vi "Test Enum.vi"(11 "Describe Variant Test in":refnum<class "Describe Variant Test.lvclass">) -> (0 "error out":errorcluster, 3 "Describe Variant Test out":refnum<class "Describe Variant Test.lvclass">)   [LabVIEW 2020, in "Describe Variant Test.lvclass"]
uses:
  Describe Variant Test.lvclass
  C:/Program Files (x86)/National Instruments/LabVIEW 2020/vi.lib/Astemes/LUnit/Test Case.lvclass
  <vilib>/Astemes/LUnit/Test Case.lvclass/Test Case.ctl
  1eb196b0-4f39-4d5f-a905-3e3c5f2415b3.vi
  <vilib>/Astemes/LUnit/Core/LUnit Test Case/Private/Append Pass Result.vi
  <vilib>/Astemes/LUnit/Core/LUnit Test Case/Private/Append Fail Result.vi
  1eb196b0-4f39-4d5f-a905-3e3c5f2415b3.vi/9c5d11cd-9439-4240-a1ee-d9baace9c924.vi
  <vilib>/Astemes/LUnit/Core/LUnit Test Case/Private/Run In UI.vi
  <vilib>/Utility/error.llb/Clear Errors.vi
  source/Framework/Utilities/Utilities.lvlib
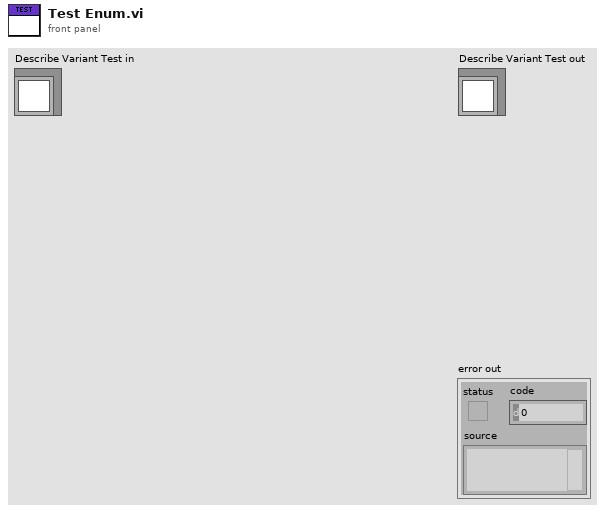
[diagram p1: front panel]
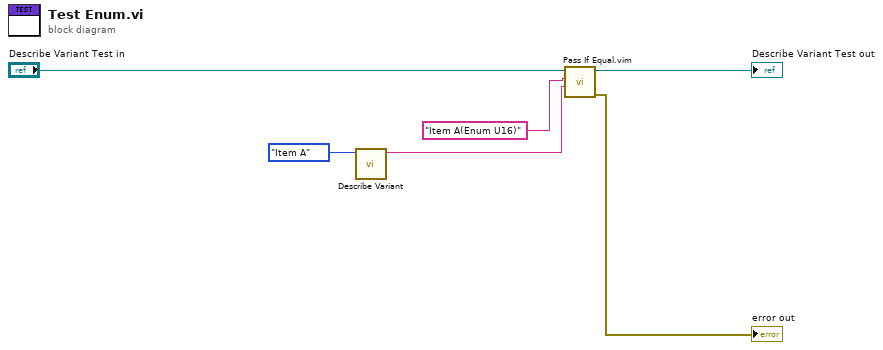
[diagram p0: block diagram]
diagram:
  n1 = call "Describe Variant.vi"("Variant"=enum16{"Item A"}."Item A") -> ("Variant Description"=w2:string)  [unwired: 8 in, 2 out]
  n2 = call "Pass If Equal.vim"("Actual"=w2, "Expected"="Item A(Enum U16)", "LUnit Test Case In"="Describe Variant Test in") -> ("error out"=→"error out":errorcluster, "LUnit Test Case Out"=→"Describe Variant Test out":refnum<class "Describe Variant Test.lvclass">)  [unwired: 7 in]
